vi "FTW-SQLite-LibraryReturnValue.vi"(0 "error in":errorcluster, 7 "Return Value":i32) -> (4 "error out":errorcluster)   [LabVIEW 2013, in "FTW-SQLite-Connector.lvclass"]
uses:
  FTW-SQLite-Connector.lvclass
panel:
  # "Inputs"
  # "Outputs"
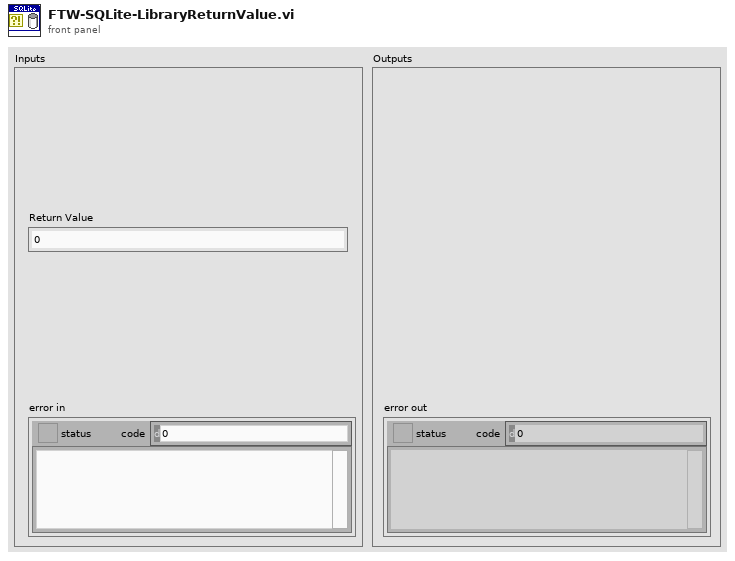
[diagram p1: front panel]
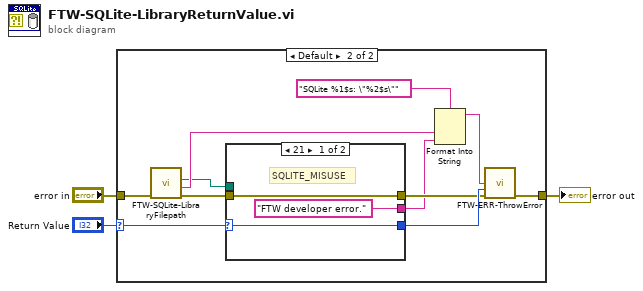
[diagram p0: block diagram]
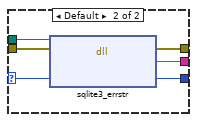
[diagram p3: hidden frame]
diagram:
  n1 = case shown="Default" "Return Value" {
    selector: "Return Value" -> [_ w5]
    tunnel: "error in" -> [w4 w15]
    tunnel: [w4 w14] -> w2
    frame 0 {
    }
    frame Default {
      n2 = call "FTW-SQLite-LibraryFilepath.vi"("error in"=w15) -> ("error out"=w10:errorcluster, "SQLite Version"=w11:string, "SQLite Library Filepath"=w6:path)  [unwired: 8 in]
      n3 = case shown="21" w5 {
        selector: w5 -> [w18 w19]
        tunnel: w10 -> [w17 w24]
        tunnel: [w18 w23] -> w9
        tunnel: [w17 w22] -> w8
        tunnel: ["FTW developer error." ("Error Message") w21] -> w7
        tunnel: w6 -> [_ w20]
        frame 21 {
          # "SQLITE_MISUSE"
        }
        frame Default {
          n4 = dll-call lib="?" fn="sqlite3_errstr"(path in=w20, error in=w24, "Error Code"=w19) -> (error out=w22:errorcluster, "Error Message"=w21:string, "Error Code"=w23:i32)  [unwired: 1 in, 1 out]
        }
      }
      n5 = Format Into String(format string="SQLite %1$s: \"%2$s\"" ("Error Message"), w11, w7) -> (resulting string=w12:string)  [unwired: 2 in, 1 out]
      n6 = call "FTW-ERR-ThrowError.vi"("Error Message"=w12, "Error Code"=w9, "error in"=w8) -> ("error out"=w14:errorcluster)  [unwired: 12 in]
    }
  }
  "error out" <- w2
